vi "PCF8574 I2C LCD Class.vi"() -> ()   [LabVIEW 2020]
uses:
  CTI-Peripheral/PCF8574 I2C LCD/PCF8574 I2C LCD.lvclass
panel:
  in  "PCF8574 I2C LCD":refnum<class "PCF8574 I2C LCD.lvclass">
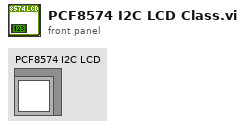
[diagram p1: front panel]
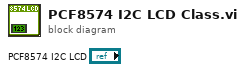
[diagram p0: block diagram]
diagram:
